vi "Write.vi"(8 "error in (no error)":errorcluster, 10 "Value":T1, 11 "Double Float.lvclass_340760 in":refnum<class "Var_EXT_1D.lvclass">) -> (0 "error out":errorcluster, 3 "Double Float.lvclass_340760 out":refnum<class "Var_EXT_1D.lvclass">)   [LabVIEW 2021, in "Var_EXT_1D.lvclass"]
uses:
  Var_EXT_1D.lvclass
  Type.ctl
  Var_EXT_1D.lvclass/Var_EXT_1D.ctl
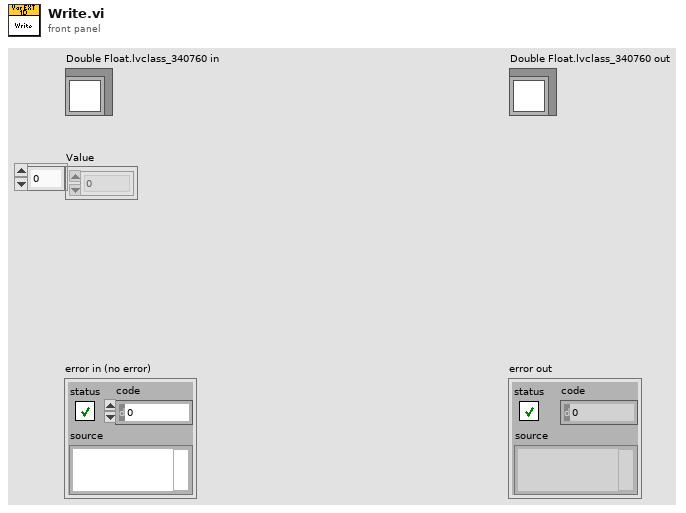
[diagram p1: front panel]
types:
  T1 = typedef "Var_EXT_1D.lvclass/Type.ctl" = ext[]
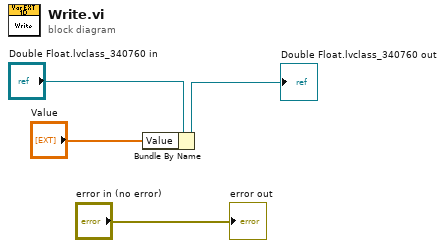
[diagram p0: block diagram]
diagram:
  n1 = Bundle By Name(cluster="Double Float.lvclass_340760 in", "Value"="Value") -> (→"Double Float.lvclass_340760 out":refnum<class "Var_EXT_1D.lvclass">)
  "error out" <- "error in (no error)"
